vi "Split Panel.vi"(8 "error in":errorcluster caption="错误输入（无错误）", 9 "VI*":refnum<vi>, 10 "Split Mode":T1, 11 "PanelDataNode 输入":refnum<class "PanelDataNode.lvclass"> caption="DNL_LabVIEW Object in") -> (0 "error out":errorcluster caption="错误输出", 2 "ChildDataNode[]":refnum<data-value>[](array[refnum]), 3 "PanelDataNode 输出":refnum<class "PanelDataNode.lvclass"> caption="DNL_LabVIEW Object out")   [LabVIEW 2016, in "PanelDataNode.lvclass"]
uses:
  PanelDataNode.lvclass
  C:/Users/CL/Desktop/ZcDAQprj0811/ZcDAQprj/Modules/DAQ-Display/PanelSplitToolkit/PanelLinkNode/PanelLinkNode.lvclass
  Split Mode.ctl
  PanelLinkNode/PanelLinkNode.lvclass/PanelLinkNode.ctl
  PanelObject/PanelObject.lvclass
  PanelLinkNode/PanelLinkNode.lvclass
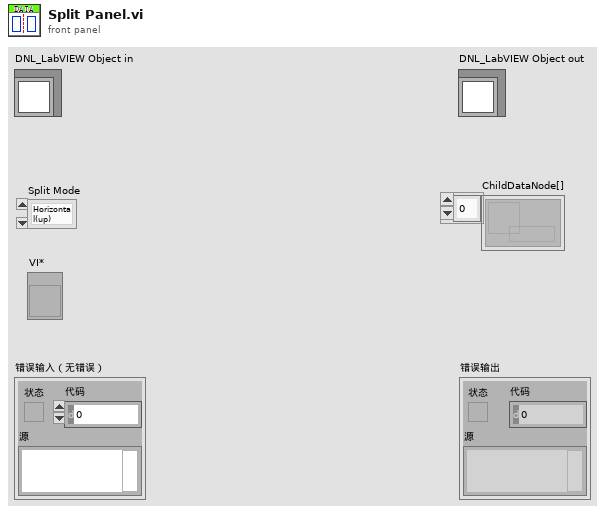
[diagram p1: front panel]
types:
  T1 = typedef "PanelDataNode.lvclass/Split Mode.ctl" = enum16{"Horizontal(up)", "Vertical(left)", "Horizontal(down)", "Vertical(right)"}
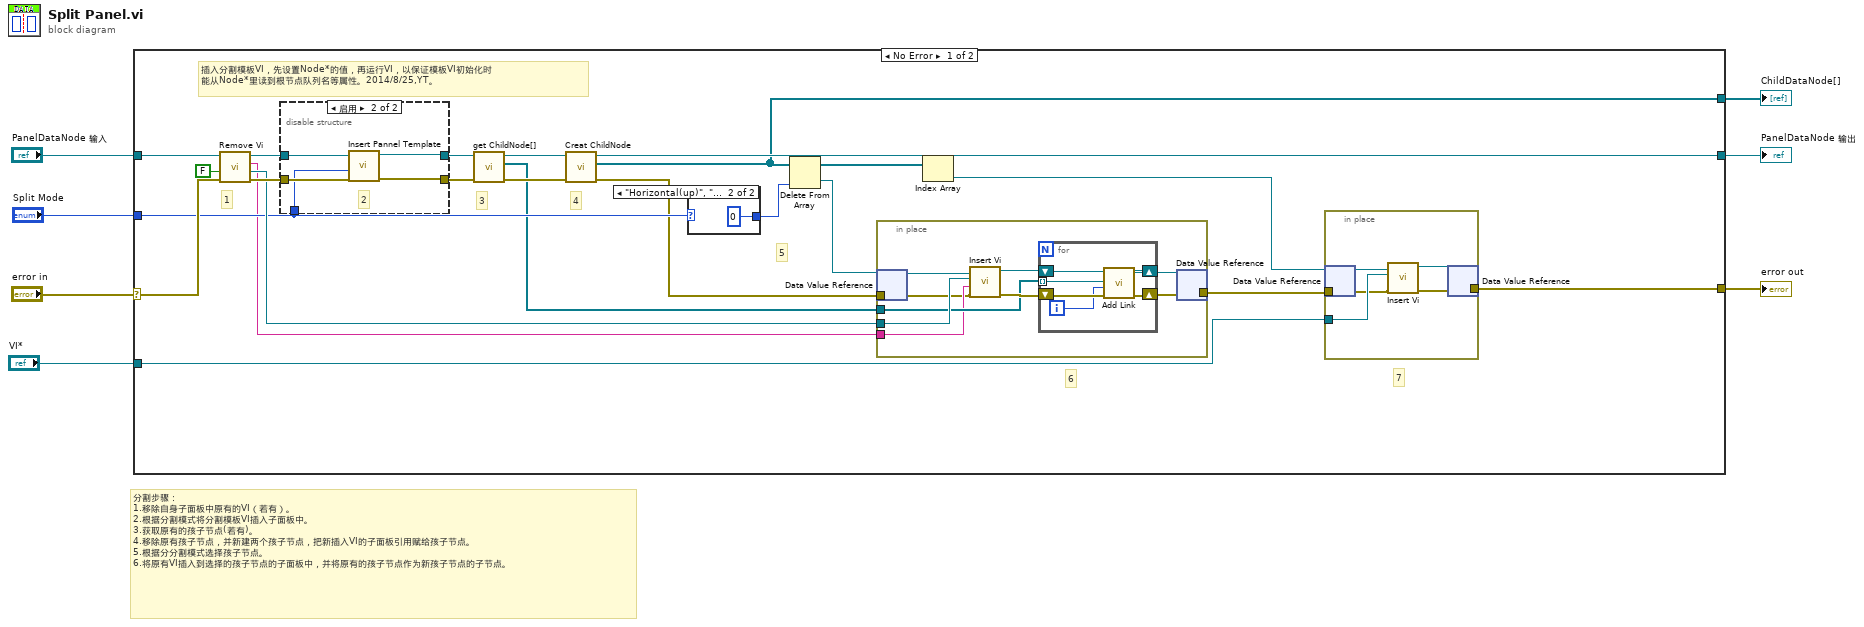
[diagram p0: block diagram]
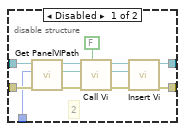
[diagram p2: hidden frame]
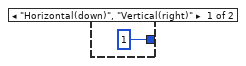
[diagram p3: hidden frame]
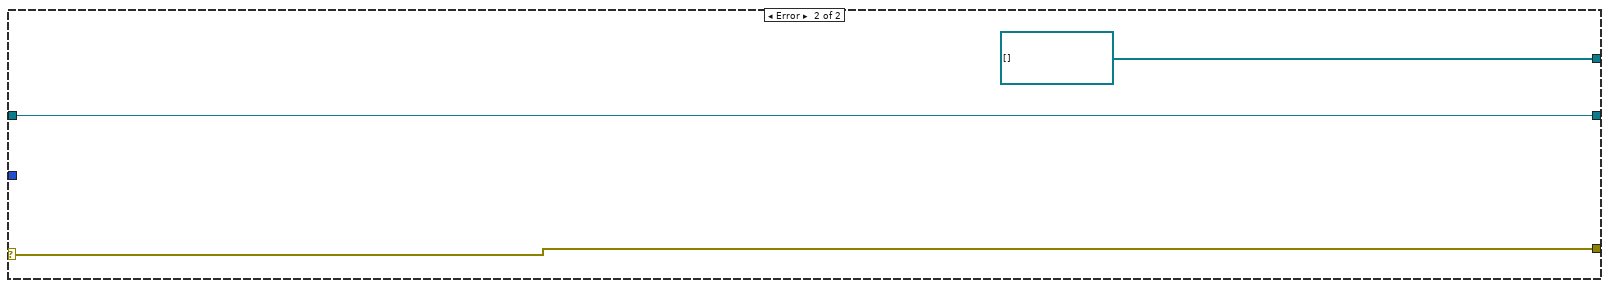
[diagram p4: hidden frame]
diagram:
  # "分割步骤：\n1.移除自身子面板中原有的VI（若有）。\n2.根据分割模式将分割模板VI插入子面板中。\n3.获取原有的孩子节点(若有)。\n4.移除原有孩子节点，并新建两个孩子节点，把新插入VI的子面板引用赋给孩子节点。\n5.根据分分割模式选择孩子节点。\n6.将原有VI插入到选择的孩子节点的子面板中，并将原有的孩子节点作为新孩子节点的子节点。"
  n1 = case shown="No Error" "error in" {
    selector: "error in" -> [w27 w72]
    tunnel: [w12 w72] -> w6
    tunnel: [w16 w71] -> w4
    tunnel: "PanelDataNode 输入" -> [w30 w71]
    tunnel: "Split Mode" -> [w19 _]
    tunnel: [w14 refnum<data-value>[] [] ("ChildDataNode[]")] -> w2
    tunnel: "VI*" -> [w8 _]
    frame No Error {
      # "7"
      # "插入分割模板VI，先设置Node*的值，再运行VI，以保证模板VI初始化时\n能从Node*里读到根节点队列名等属性。2014/8/25,YT。"
      # "6"
      # "5"
      # "4"
      # "3"
      # "1"
      n2 = call-dynamic "Remove Vi.vi"("error in"=w27, "Abort VI"=FALSE, "PanelDataNode 输入"=w30) -> ("error out"=w28:errorcluster, "VI*"=w25:refnum<vi>, "ViValue"=w15:string, "PanelDataNode 输出"=w29:refnum<class "PanelDataNode.lvclass">)  [unwired: 5 in]
      n3 = disable-structure shown="启用" {
        disable-tunnel: w29 -> [w47 w52]
        disable-tunnel: w28 -> [w46 w50]
        disable-tunnel: [w45 w51] -> w24
        disable-tunnel: [w44 w49] -> w23
        disable-tunnel: w19 -> [w43 w48]
        frame Disabled {
          # "2"
          n4 = call-dynamic "Get PanelVIPath.vi"("error in (no error)"=w46, "Split Mode"=w43, "PanelDataNode 输入"=w47) -> ("error out"=w40:errorcluster, "panel path"=w37:path, "PanelDataNode 输出"=w42:refnum<class "PanelDataNode.lvclass">)  [unwired: 4 in]
          n5 = call-dynamic "Call Vi.vi"("Auto Dispose Ref"=FALSE, "error in (no error)"=w40, "Vi Path"=w37, "PanelDataNode 输入"=w42) -> ("error out"=w39:errorcluster, "VI*"=w38:refnum<vi>, "PanelDataNode 输出"=w41:refnum<class "PanelDataNode.lvclass">)  [unwired: 5 in]
          n6 = call-dynamic "Insert Vi.vi"("error in (no error)"=w39, "VI*"=w38, "PanelDataNode 输入"=w41) -> ("error out"=w44:errorcluster, "PanelDataNode 输出"=w45:refnum<class "PanelDataNode.lvclass">)  [unwired: 7 in]
        }
        frame Enabled {
          # "2"
          n7 = call "Insert Pannel Template.vi"("error in"=w50, "Split Mode"=w48, "PanelDataNode in"=w52) -> ("error out"=w49:errorcluster, "PanelDataNode out"=w51:refnum<class "PanelDataNode.lvclass">)  [unwired: 7 in]
        }
      }
      n8 = call "get ChildNode[].vi"("error in (no error)"=w23, "PanelLinkNode输入"=w24) -> ("error out"=w20:errorcluster, "ChildNode*[]"=w9:refnum<data-value>[], "PanelLinkNode输出"=w21:refnum<class "PanelDataNode.lvclass">)  [unwired: 7 in]
      n9 = call-dynamic "Creat ChildNode.vi"("error in"=w20, "ParentDataNode in"=w21) -> ("error out"=w18:errorcluster, "ChildDataNode[]"=w14:refnum<data-value>[], "ParentDataNode out"=w16:refnum<class "PanelDataNode.lvclass">)  [unwired: 7 in]
      n10 = case shown="\"Horizontal(up)\", \"Vertical(left)\", Default" w19 {
        tunnel: [1 0] -> w17
        frame "Horizontal(down)", "Vertical(right)" {
        }
        frame "Horizontal(up)", "Vertical(left)", Default {
        }
      }
      n11 = Delete From Array(array=w14, index=w17) -> (deleted portion=w22:refnum<data-value>, array with subset deleted=w11:refnum<data-value>[])  [unwired: 1 in]
      n12 = in-place {
        in-place-border: w18 -> [w55]
        in-place-border: w25 -> [w63]
        in-place-border: w9 -> [w59]
        in-place-border: [w58] -> w13
        in-place-border: w15 -> [w57]
        n13 = in-place-dvr #1(w22) -> (w56:refnum<class "PanelDataNode.lvclass">)  [unwired: 1 out]
        n14 = call-dynamic "Insert Vi.vi"("error in (no error)"=w55, "ViValue"=w57, "VI*"=w63, "PanelDataNode 输入"=w56) -> ("error out"=w60:errorcluster, "PanelDataNode 输出"=w62:refnum<class "PanelDataNode.lvclass">)  [unwired: 6 in]
        n15 = for {
          shift-right: [w68] -> w61
          shift-left: w62 -> [w69]
          tunnel: w59 -> [w64] mode=indexing
          shift-right: [w66] -> w58
          shift-left: w60 -> [w67]
          i -> [w65]
          n16 = call-dynamic "Add Link.vi"("ParentLinkNode in"=w69, "ChildNode* in"=w64, "L\\R Child"=w65, "error in (no error)"=w67) -> ("ParentLinkNode out"=w68:refnum<class "PanelDataNode.lvclass">, "error out"=w66:errorcluster)  [unwired: 5 in]
        }
        n17 = in-place-dvr #1(w61) -> ()  [unwired: 2 out]
      }
      n18 = Index Array(array=w11) -> (element=w10:refnum<data-value>)  [unwired: 1 in]
      n19 = in-place {
        in-place-border: w13 -> [w33]
        in-place-border: w8 -> [w35]
        in-place-border: [w32] -> w12
        n20 = in-place-dvr #2(w10) -> (w34:refnum<class "PanelDataNode.lvclass">)  [unwired: 1 out]
        n21 = call-dynamic "Insert Vi.vi"("error in (no error)"=w33, "VI*"=w35, "PanelDataNode 输入"=w34) -> ("error out"=w32:errorcluster, "PanelDataNode 输出"=w31:refnum<class "PanelDataNode.lvclass">)  [unwired: 7 in]
        n22 = in-place-dvr #2(w31) -> ()  [unwired: 2 out]
      }
    }
    frame Error {
    }
  }
  "error out" <- w6
  "PanelDataNode 输出" <- w4
  "ChildDataNode[]" <- w2
